vi "Read record from DB.vi"(8 "error in (no error)":errorcluster, 10 "Record":T1, 11 "Interface Elevator in":refnum<class "Interface Elevator.lvclass">) -> (0 "error out":errorcluster, 3 "Interface Elevator out":refnum<class "Interface Elevator.lvclass">)   [LabVIEW 2022 SP3, in "Interface Elevator.lvclass"]
uses:
  Interface Elevator.lvclass
  Configuration Database Actor/Configuration Database Actor/Record -Cluster.ctl
  Configuration Database Actor/Configuration Database Actor/Configuration Database Actor.lvclass
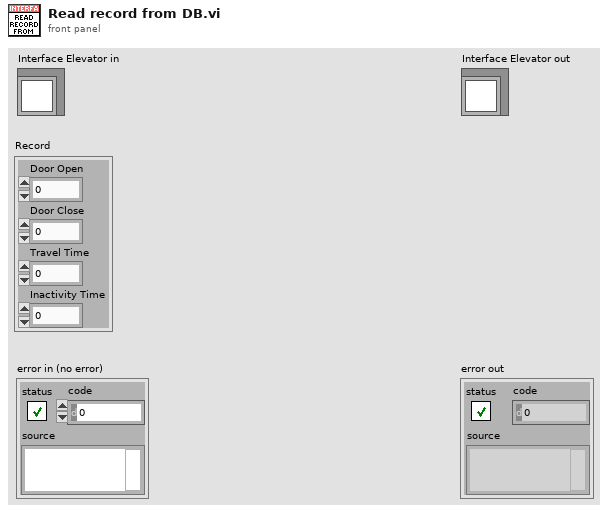
[diagram p1: front panel]
types:
  T1 = typedef "Configuration Database Actor.lvlib/Configuration Database Actor.lvclass/Record -Cluster.ctl" = cluster{"Door Open":dbl, "Door Close":dbl, "Travel Time":dbl, "Inactivity Time":dbl}
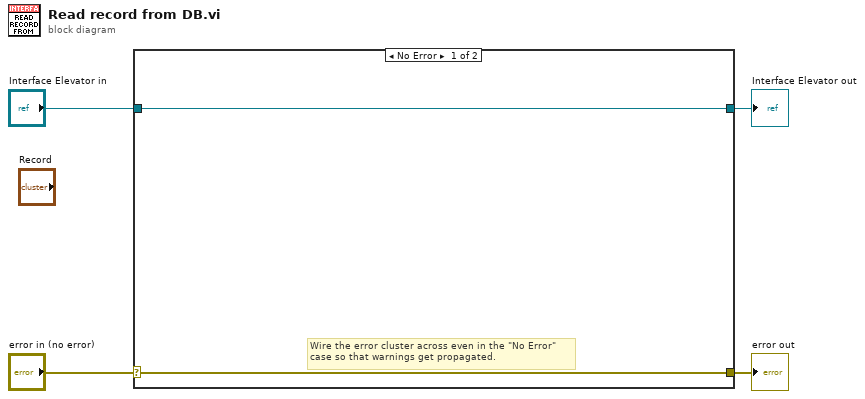
[diagram p0: block diagram]
diagram:
  n1 = case shown="No Error" "error in (no error)" {
    selector: "error in (no error)" -> [w5 w8]
    tunnel: [w5 w8] -> w3
    tunnel: [w6 w7] -> w1
    tunnel: "Interface Elevator in" -> [w6 w7]
    frame No Error {
      # "Wire the error cluster across even in the \"No Error\"\ncase so that warnings get propagated."
    }
    frame Error {
    }
  }
  "error out" <- w3
  "Interface Elevator out" <- w1
